vi "s3_plot.vi"() -> ()   [LabVIEW 2018]
uses:
  <vilib>/AWS Toolkit/Core/HTTP Request/AWS Credentials.ctl
  <vilib>/AWS Toolkit/S3/PUT Object Request Parameters.ctl
  <vilib>/AWS Toolkit/S3/ACL.ctl
  <vilib>/AWS Toolkit/S3/Storage Class.ctl
  <vilib>/AWS Toolkit/Core/HTTP Request/Name Value Pair.ctl
  <vilib>/AWS Toolkit/Core/HTTP Request/HTTP Request.lvclass
  <vilib>/AWS Toolkit/S3/Bucket/Bucket.lvclass
  <vilib>/AWS Toolkit/S3/NI_AWS_S3.lvlib
panel:
  out "appended path":path
  out "size(s)":i32
  out "XY Graph":cluster{dbl[], dbl[]}(graph)
  out "Data":string
  in  "Bucket Name":string
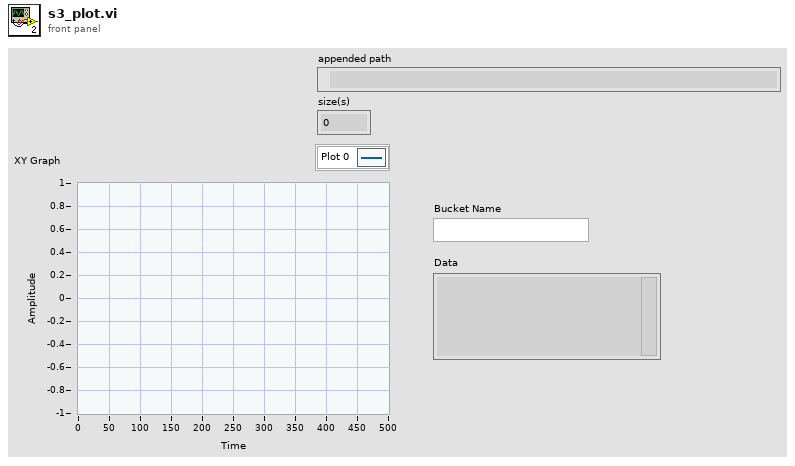
[diagram p1: front panel]
types:
  T1 = typedef "NI_AWS_Core.lvlib/HTTP Request.lvclass/AWS Credentials.ctl" = cluster{"Access Key":string, "Secret Key":string}
  T2 = typedef "NI_AWS_S3.lvlib/Object Content.ctl" = cluster{"Key":string, "Last Modified":timestamp, "ETag":string, "Size":u64, "Storage Class":T3, "Owner":T4}
  T3 = typedef "NI_AWS_S3.lvlib/Storage Class.ctl" = enum16{"STANDARD", "REDUCED_REDUNDANCY"}
  T4 = typedef "NI_AWS_S3.lvlib/Owner.ctl" = cluster{"ID":string, "Display Name":string}
  T5 = typedef "NI_AWS_S3.lvlib/PUT Object Request Parameters.ctl" = cluster{"Content Type":string, "ACL":T6, "Storage Class":T3, "User-Defined Metadata":T7[]}
  T6 = typedef "NI_AWS_S3.lvlib/ACL.ctl" = enum16{"private", "public-read", "public-read-write", "aws-exec-read", "authenticated-read", "bucket-owner-read", "bucket-owner-full-control"}
  T7 = typedef "NI_AWS_Core.lvlib/HTTP Request.lvclass/Name Value Pair.ctl" = cluster{"name":string, "value":string}
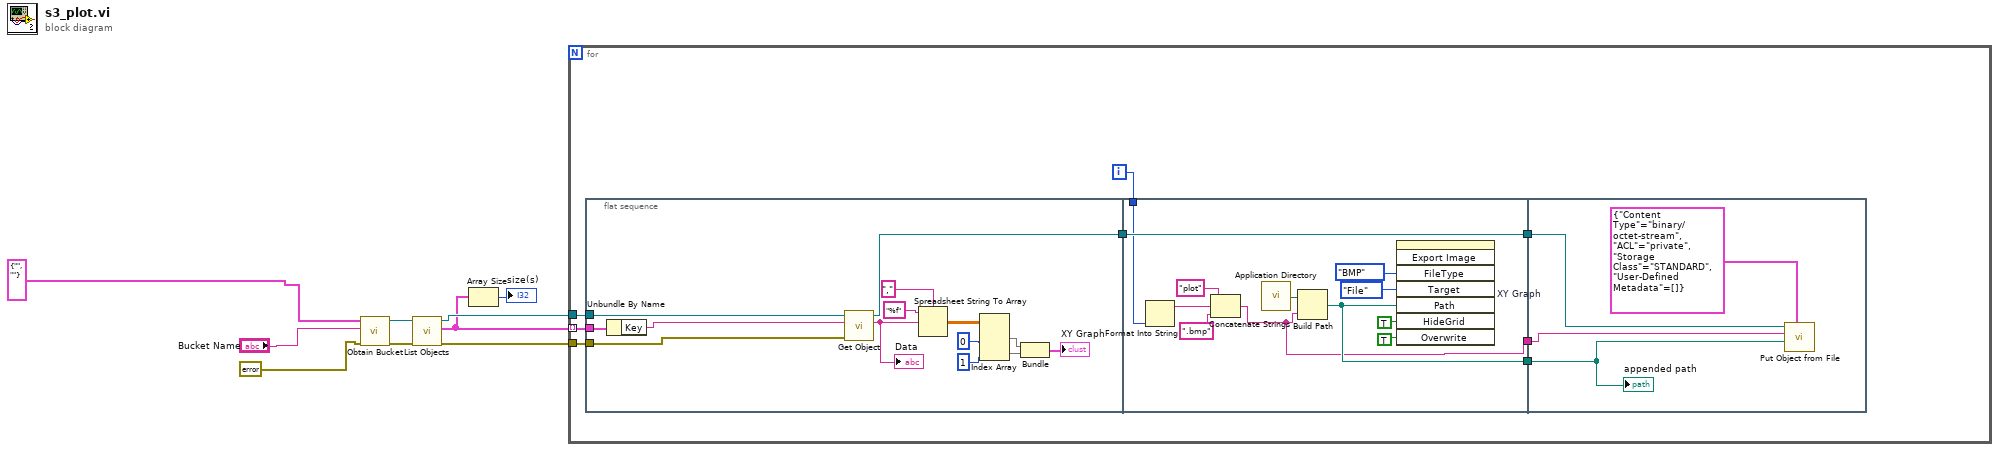
[diagram p0: block diagram]
diagram:
  n1 = call <vilib>:"Obtain Bucket.vi"("error in (no error)"=errorcluster {"status"=FALSE, "code"=0, "source"=""} ("error constant"), "Bucket name"="Bucket Name", "AWS Credentials"=T1 {"Access Key"="", "Secret Key"=""}) -> ("error out"=w6:errorcluster, "Bucket"=w7:refnum<class "Bucket.lvclass">)  [unwired: 7 in]
  n2 = call <vilib>:"List Objects.vi"("error in (no error)"=w6, "Bucket in"=w7) -> ("error out"=w1:errorcluster, "Objects"=w2:T2[], "Bucket out"=w3:refnum<class "Bucket.lvclass">)  [unwired: 6 in, 1 out]
  n3 = Array Size(array=w2) -> (size(s)=→"size(s)":i32)
  n4 = for {
    tunnel: w3 -> [w17]
    tunnel: w2 -> [w16] mode=indexing
    tunnel: w1 -> [w15]
    i -> [w11]
    n5 = flat-sequence {
      tunnel: w17 -> [w22]
      tunnel: w16 -> [w21]
      tunnel: w15 -> [w20]
      tunnel: [w19] -> w13
      tunnel: [w35] -> w14
      tunnel: w13 -> [w35]
      tunnel: [w34] -> w12
      tunnel: w11 -> [w33]
      tunnel: [w32] -> w10
      tunnel: w14 -> [w47]
      tunnel: w12 -> [w46]
      tunnel: w10 -> [w44]
      frame #0 {
        n6 = Unbundle By Name(w21) -> ("Key"=w18:string)
        n7 = call <vilib>:"Get Object.vi"("error in (no error)"=w20, "Object Path"=w18, "Bucket in"=w22) -> ("Data"=w27:string, "Bucket out"=w19:refnum<class "Bucket.lvclass">)  [unwired: 4 in, 3 out]
        "Data" <- w27
        n8 = Spreadsheet String To Array(delimiter (Tab)=",", format string="%f", spreadsheet string=w27) -> (array=w28:dbl[][])  [unwired: 1 in]
        n9 = Index Array(array=w28, index (col) #1=0 ("disabled index (col)"), index (col) #2=1 ("index (col)")) -> (element #1=w30:dbl[], element #2=w31:dbl[])  [unwired: 2 in]
        n10 = Bundle(w30, w31) -> (→"XY Graph":cluster{dbl[], dbl[]})  [unwired: 1 in]
      }
      frame #1 {
        n11 = Format Into String(w33) -> (resulting string=w37:string)  [unwired: 3 in, 1 out]
        n12 = Concatenate Strings("plot" ("string"), w37, ".bmp" ("string")) -> (w32:string)
        n13 = call <vilib>:"Application Directory.vi"() -> ("Application Directory"=w36:path)
        n14 = Build Path(base path=w36, name or relative path=w32) -> (appended path=w34:path)
        n15 = invoke on="XY Graph" class="XYGraph (strict)" method="Export Image"("FileType"=enum32{"BMP", "EPS", "EMF", "PICT"}."BMP" ("File Type"), "Target"=enum32{"File", "Clipboard"}."File", "Path"=w34, "HideGrid"=TRUE ("Hide Grid"), "Overwrite"=TRUE ("Always Overwrite")) -> ()  [unwired: 3 in, 8 out]
      }
      frame #2 {
        n16 = call <vilib>:"Put Object from File.vi"("Object Parameters"=T5 {"Content Type"="binary/octet-stream", "ACL"=enum."private", "Storage Class"=enum."STANDARD", "User-Defined Metadata"=[]}, "File"=w46, "Object Path"=w44, "Bucket in"=w47) -> ()  [unwired: 3 in, 5 out]
        "appended path" <- w46
      }
    }
  }
